vi "BRig_RT__Case_Idle__State_Cue.vi"(4 "input_cLick_R_prev":u32, 6 "input_cLick_R":u32, 7 "input_state":T1=enum."DispenseWater_pre", 8 "input_cLick_L_prev":u32, 9 "input_cLick_L":u32, 11 "input_dataMTrig":u16[](array[numeric])) -> (3 "output_dataMTrig":u16[](array[numeric]), 5 "output_state":T1)   [LabVIEW 2014]
uses:
  myRIO_BRig_RT__Case_NonExp_stateList.ctl
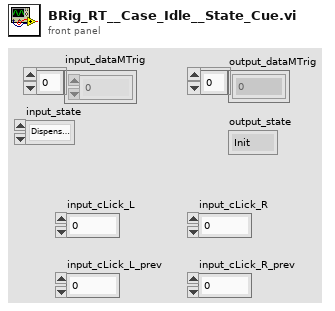
[diagram p1: front panel]
types:
  T1 = typedef "myRIO_BRig_RT__Case_NonExp_stateList.ctl" = enum16{"Init", "UploadSettings_pre", "UploadSettings_Read_dataExp", "UploadSettings_dataExp_1", "UploadSettings_dataExp_2", "UploadSettings_Read_dataLC", "UploadSettings_dataLC_1", "UploadSettings_dataLC_2", "UploadSettings_dataLC_3", "UploadSettings_dataLC_4", "UploadSettings_Read_dataMTrig", "UploadSettings_dataMTrig_1", "UploadSettings_post", "Idle_pre", "IdleEmpty", "IdleEmpty2", "IdleEmpty3", "IdleEmpty4", "Idle", "Idle_2", "Idle_3", "Idle_4", "Idle_5", "Idle_6", "Idle_post", "Cue_pre__pre", "Cue_pre", "Cue", "Cue_LED", "Cue_post", "RewardCalibration_pre", "RewardCalibration", "DispenseWater_pre__pre", "DispenseWater_pre", "DispenseWater", "DispenseWater_post", "TestConnection", "SendData", "Get_FPGA_count_per_ms", "End", "commTCP_connect"}
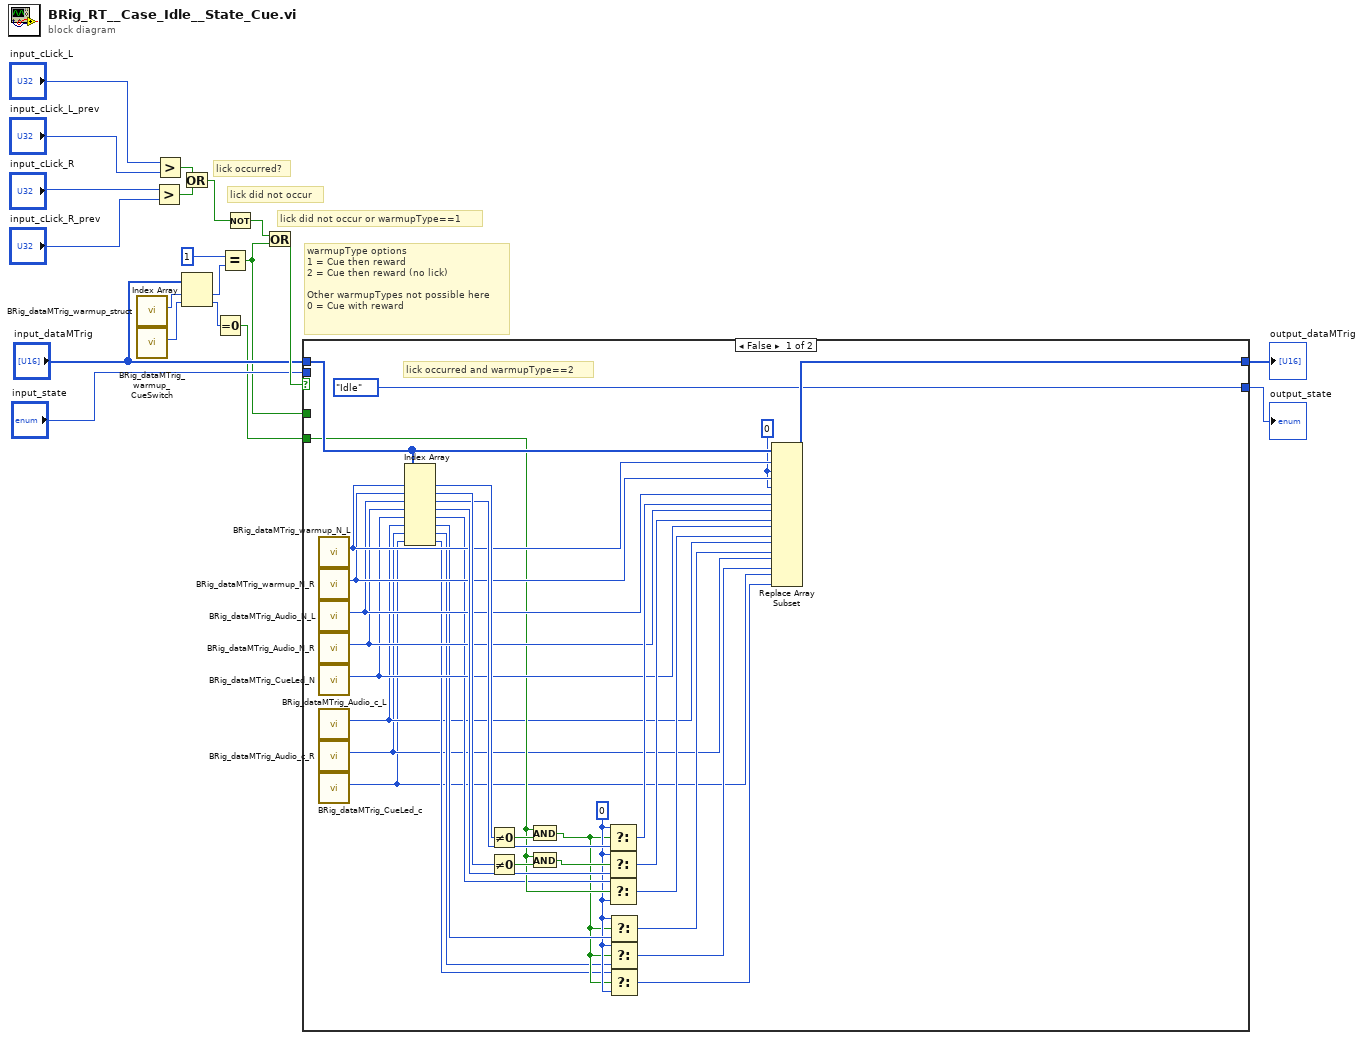
[diagram p0: block diagram]
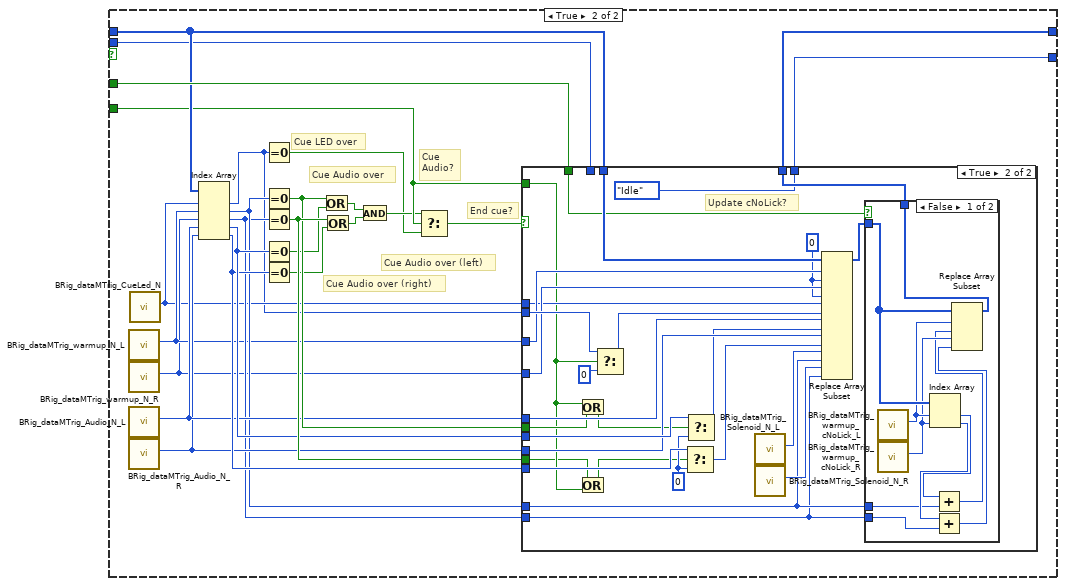
[diagram p2: hidden frame]
diagram:
  # "lick did not occur"
  # "warmupType options\n1 = Cue then reward\n2 = Cue then reward (no lick)\n\nOther warmupTypes not possible here\n0 = Cue with reward"
  # "lick did not occur or warmupType==1"
  # "lick occurred?"
  n1 = call "BRig_dataMTrig_warmup_struct.vi"() -> ("output_warmup_struct"=w15:i32)  [unwired: 11 in]
  n2 = call "BRig_dataMTrig_warmup_CueSwitch.vi"() -> ("output_warmup_CueSwitch"=w3:i32)  [unwired: 11 in]
  n3 = Greater?(x="input_cLick_R", y="input_cLick_R_prev") -> (0:w20:bool)
  n4 = Greater?(x="input_cLick_L", y="input_cLick_L_prev") -> (0:w19:bool)
  n5 = Or(x=w19, y=w20) -> (x .or. y?=w18:bool)
  n6 = Index Array(array="input_dataMTrig", index #1=w15, index #2=w3) -> (element #1=w13:u16, element #2=w2:u16)
  n7 = Equal To 0?(x=w2) -> (x = 0?=w1:bool)
  n8 = Equal?(x=u16 1 ("y"), y=w13) -> (x = y?=w8:bool)
  n9 = Not(x=w18) -> (.not. x?=w17:bool)
  n10 = Or(x=w17, y=w8) -> (x .or. y?=w16:bool)
  n11 = case shown="False" w16 {
    tunnel: "input_dataMTrig" -> [w50 w76]
    tunnel: [w52 w75] -> w11
    tunnel: "input_state" -> [_ w74]
    tunnel: [myRIO_BRig_RT__Case_NonExp_stateList."Idle" ("t") w62] -> w10
    tunnel: w8 -> [_ w77]
    tunnel: w1 -> [w34 w57]
    frame False {
      w30 = u16 0 ("new element/subarray")
      w39 = u16 0 ("new element/subarray")
      # "lick occurred and warmupType==2"
      n12 = call "BRig_dataMTrig_warmup_N_L.vi"() -> ("output_warmup_N_L"=w45:i32)  [unwired: 11 in]
      n13 = call "BRig_dataMTrig_warmup_N_R.vi"() -> ("output_warmup_N_R"=w44:i32)  [unwired: 11 in]
      n14 = call "BRig_dataMTrig_Audio_N_L.vi"() -> ("output_Audio_N_L"=w43:i32)  [unwired: 11 in]
      n15 = call "BRig_dataMTrig_Audio_N_R.vi"() -> ("output_Audio_N_R"=w40:i32)  [unwired: 11 in]
      n16 = call "BRig_dataMTrig_CueLed_N.vi"() -> ("output_CueLed_N"=w35:i32)  [unwired: 11 in]
      n17 = call "BRig_dataMTrig_Audio_c_L.vi"() -> ("output_Audio_c_L"=w25:i32)  [unwired: 11 in]
      n18 = call "BRig_dataMTrig_Audio_c_R.vi"() -> ("output_Audio_c_R"=w24:i32)  [unwired: 11 in]
      n19 = call "BRig_dataMTrig_CueLed_c.vi"() -> ("output_CueLed_c"=w22:i32)  [unwired: 11 in]
      n20 = Index Array(array=w50, index #1=w45, index #2=w44, index #3=w43, index #4=w40, index #5=w35, index #6=w25, index #7=w24, index #8=w22) -> (element #1=w49:u16, element #2=w48:u16, element #3=w47:u16, element #4=w46:u16, element #5=w31:u16, element #6=w32:u16, element #7=w28:u16, element #8=w27:u16)
      n21 = Not Equal To 0?(x=w49) -> (x != 0?=w38:bool)
      n22 = Not Equal To 0?(x=w48) -> (x != 0?=w37:bool)
      n23 = And(x=w34, y=w38) -> (x .and. y?=w29:bool)
      n24 = And(x=w34, y=w37) -> (x .and. y?=w36:bool)
      n25 = Select(t=w30, s=w29, f=w47) -> (s? t:f=w42:u16)
      n26 = Select(t=w30, s=w36, f=w46) -> (s? t:f=w41:u16)
      n27 = Select(t=w31, s=w34, f=w30) -> (s? t:f=w33:u16)
      n28 = Select(t=w30, s=w29, f=w32) -> (s? t:f=w26:u16)
      n29 = Select(t=w30, s=w29, f=w28) -> (s? t:f=w23:u16)
      n30 = Select(t=w27, s=w29, f=w30) -> (s? t:f=w21:u16)
      n31 = Replace Array Subset(array=w50, new element #1=w39, index #1=w45, new element #2=w39, index #2=w44, new element #3=w42, index #3=w43, new element #4=w41, index #4=w40, new element #5=w33, index #5=w35, new element #6=w26, index #6=w25, new element #7=w23, index #7=w24, new element #8=w21, index #8=w22) -> (w52:u16[])
    }
    frame True {
      # "Cue Audio over"
      # "Cue Audio over (right)"
      # "Cue Audio over (left)"
      # "Cue LED over"
      # "Cue\nAudio?"
      # "End cue?"
      n32 = call "BRig_dataMTrig_warmup_N_L.vi"() -> ("output_warmup_N_L"=w65:i32)  [unwired: 11 in]
      n33 = call "BRig_dataMTrig_warmup_N_R.vi"() -> ("output_warmup_N_R"=w64:i32)  [unwired: 11 in]
      n34 = call "BRig_dataMTrig_Audio_N_L.vi"() -> ("output_Audio_N_L"=w69:i32)  [unwired: 11 in]
      n35 = call "BRig_dataMTrig_Audio_N_R.vi"() -> ("output_Audio_N_R"=w68:i32)  [unwired: 11 in]
      n36 = call "BRig_dataMTrig_CueLed_N.vi"() -> ("output_CueLed_N"=w63:i32)  [unwired: 11 in]
      n37 = Index Array(array=w76, index #1=w63, index #2=w65, index #3=w64, index #4=w69, index #5=w68) -> (element #1=w53:u16, element #2=w67:u16, element #3=w66:u16, element #4=w71:u16, element #5=w70:u16)
      n38 = Equal To 0?(x=w53) -> (x = 0?=w54:bool)
      n39 = Equal To 0?(x=w67) -> (x = 0?=w72:bool)
      n40 = Equal To 0?(x=w66) -> (x = 0?=w73:bool)
      n41 = Equal To 0?(x=w71) -> (x = 0?=w60:bool)
      n42 = Equal To 0?(x=w70) -> (x = 0?=w61:bool)
      n43 = Or(x=w72, y=w60) -> (x .or. y?=w59:bool)
      n44 = Or(x=w73, y=w61) -> (x .or. y?=w58:bool)
      n45 = And(x=w59, y=w58) -> (x .and. y?=w56:bool)
      n46 = Select(t=w56, s=w57, f=w54) -> (s? t:f=w55:bool)
      n47 = case shown="True" w55 {
        tunnel: w77 -> [_ w102]
        tunnel: w76 -> [w79 w107]
        tunnel: [w79 w100] -> w75
        tunnel: w74 -> [w78 _]
        tunnel: w57 -> [_ w85]
        tunnel: w73 -> [_ w84]
        tunnel: w72 -> [_ w87]
        tunnel: w71 -> [_ w106]
        tunnel: w70 -> [_ w105]
        tunnel: w69 -> [_ w104]
        tunnel: w68 -> [_ w103]
        tunnel: w67 -> [_ w81]
        tunnel: w66 -> [_ w80]
        tunnel: w65 -> [_ w93]
        tunnel: w64 -> [_ w92]
        tunnel: w63 -> [_ w90]
        tunnel: [w78 myRIO_BRig_RT__Case_NonExp_stateList."Idle" ("t")] -> w62
        tunnel: w53 -> [_ w95]
        frame False {
        }
        frame True {
          w98 = u16 0 ("f")
          w91 = u16 0 ("new element/subarray")
          # "Update cNoLick?"
          n48 = Or(x=w85, y=w87) -> (x .or. y?=w88:bool)
          n49 = Or(x=w84, y=w85) -> (x .or. y?=w86:bool)
          n50 = Select(t=w95, s=w85, f=u16 0) -> (s? t:f=w89:u16)
          n51 = Select(t=w105, s=w86, f=w98) -> (s? t:f=w96:u16)
          n52 = Select(t=w106, s=w88, f=w98) -> (s? t:f=w97:u16)
          n53 = call "BRig_dataMTrig_Solenoid_N_L.vi"() -> ("output_Solenoid_N_L"=w83:i32)  [unwired: 11 in]
          n54 = call "BRig_dataMTrig_Solenoid_N_R.vi"() -> ("output_Solenoid_N_R"=w82:i32)  [unwired: 11 in]
          n55 = Replace Array Subset(array=w107, new element #1=w91, index #1=w93, new element #2=w91, index #2=w92, new element #3=w89, index #3=w90, new element #4=w97, index #4=w104, new element #5=w96, index #5=w103, new element #6=w81, index #6=w83, new element #7=w80, index #7=w82) -> (w101:u16[])
          n56 = case shown="False" w102 {
            tunnel: w101 -> [w113 w118]
            tunnel: [w112 w118] -> w100
            tunnel: w81 -> [w115 _]
            tunnel: w80 -> [w114 _]
            frame False {
              n57 = call "BRig_dataMTrig_warmup_cNoLick_L.vi"() -> ("output_warmup_cNoLick_L"=w111:i32)  [unwired: 11 in]
              n58 = call "BRig_dataMTrig_warmup_cNoLick_R.vi"() -> ("output_warmup_cNoLick_R"=w110:i32)  [unwired: 11 in]
              n59 = Index Array(array=w113, index #1=w111, index #2=w110) -> (element #1=w116:u16, element #2=w117:u16)
              n60 = Add(x=w116, y=w115) -> (x+y=w109:u16)
              n61 = Add(x=w117, y=w114) -> (x+y=w108:u16)
              n62 = Replace Array Subset(array=w113, new element #1=w109, index #1=w111, new element #2=w108, index #2=w110) -> (w112:u16[])
            }
            frame True {
            }
          }
        }
      }
    }
  }
  "output_dataMTrig" <- w11
  "output_state" <- w10
